vi "smff-calc-rate.vi"(8 "Time pass through":dbl=-1.0, 11 "Value":dbl) -> (3 "Value Rate":dbl)   [LabVIEW 2019]
uses:
  <vilib>/Utility/semaphor.llb/Obtain Semaphore Reference.vi
  <vilib>/Rock Robotics/WPI/ThirdParty/JAS_Junk/TrajLib/Timer_Reset.vi
  <vilib>/Rock Robotics/WPI/ThirdParty/JAS_Junk/TrajLib/Trajectory_Library.lvlib
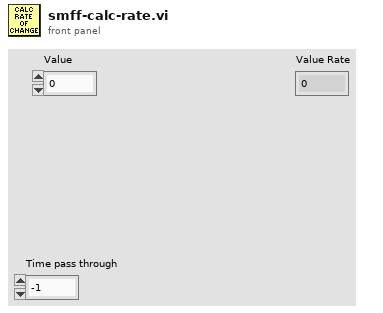
[diagram p1: front panel]
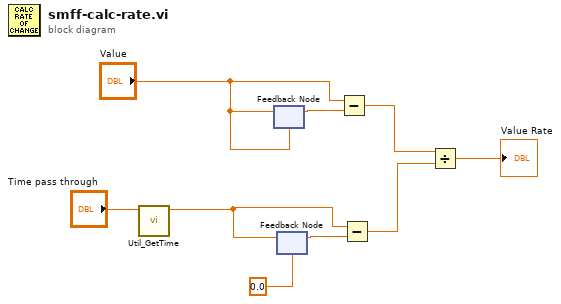
[diagram p0: block diagram]
diagram:
  n1 = call <vilib>:"Util_GetTime.vi"("Pass_Through_Time"="Time pass through") -> ("FPGA_Time_Seconds"=w5:dbl)  [unwired: 9 in, 1 out]
  n2 = feedback #1("Value") -> (w8:dbl)
  n3 = feedback-in #1("Value") -> ()
  n4 = feedback #2(0.0 ("FPGA_Time_Seconds")) -> (w6:dbl)
  n5 = feedback-in #2(w5) -> ()
  n6 = Subtract(x="Value", y=w8) -> (x-y=w3:dbl)
  n7 = Subtract(x=w5, y=w6) -> (x-y=w2:dbl)
  n8 = Divide(x=w3, y=w2) -> (x/y=→"Value Rate":dbl)
